vi "get_image_path.vi"(11 "Image directory/path":path) -> (2 "Init image index":u32, 3 "Image path array":path[](array[path]))   [LabVIEW 2024]
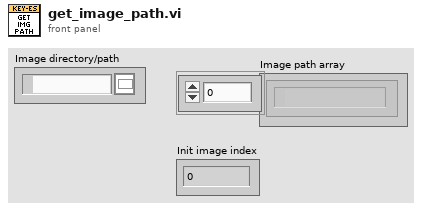
[diagram p1: front panel]
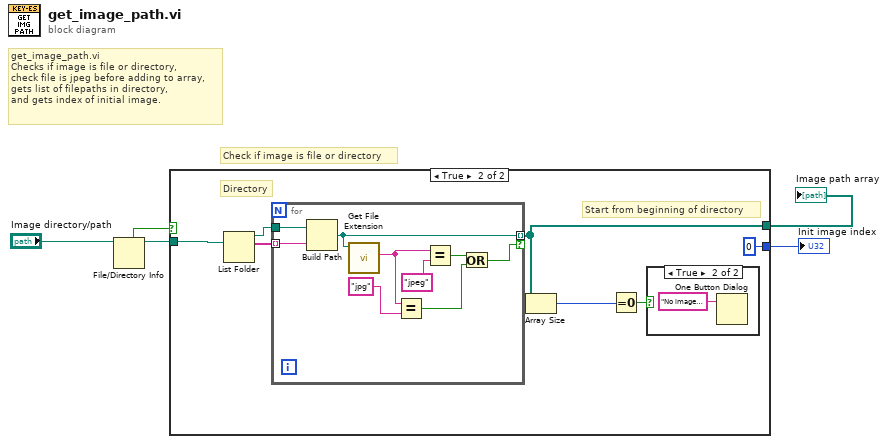
[diagram p0: block diagram]
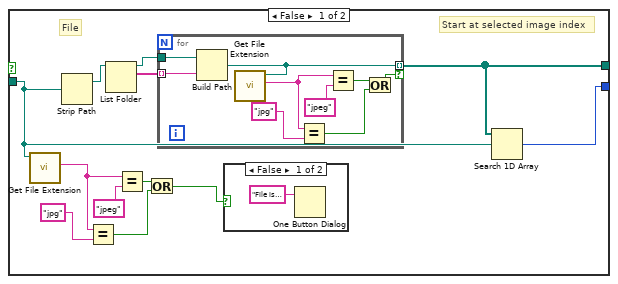
[diagram p2: hidden frame]
diagram:
  # "get_image_path.vi\nChecks if image is file or directory,\ncheck file is jpeg before adding to array,\ngets list of filepaths in directory,\nand gets index of initial image."
  # "Check if image is file or directory"
  n1 = File/Directory Info(path="Image directory/path") -> (path out=w4:path, directory=w5:bool)  [unwired: 1 in, 5 out]
  n2 = case shown="True" w5 {
    tunnel: w4 -> [w14 w34]
    tunnel: [w13 w30] -> w2
    tunnel: [w12 u32 0 ("millisecond multiple")] -> w1
    frame False {
      # "File"
      # "Start at selected image index"
      n3 = call <vilib>:"Get File Extension.vi"("file"=w14) -> ("lowercase file extension"=w7:string)  [unwired: 6 in, 4 out]
      n4 = Strip Path(path=w14) -> (stripped path=w15:path)  [unwired: 1 out]
      n5 = Equal?(x=w7, y="jpg") -> (x = y?=w9:bool)
      n6 = List Folder(path=w15) -> (path out=w16:path, filenames=w17:string[])  [unwired: 3 in, 2 out]
      n7 = Equal?(x=w7, y="jpeg") -> (x = y?=w10:bool)
      n8 = Or(x=w10, y=w9) -> (x .or. y?=w6:bool)
      n9 = for {
        tunnel: w17 -> [w25] mode=indexing
        tunnel: w16 -> [w26]
        tunnel: [w24] -> w13 mode=indexing if=w18
        n10 = Build Path(base path=w26, name or relative path=w25) -> (appended path=w24:path)
        n11 = call <vilib>:"Get File Extension.vi"("file"=w24) -> ("lowercase file extension"=w19:string)  [unwired: 6 in, 4 out]
        n12 = Equal?(x=w19, y="jpg") -> (x = y?=w21:bool)
        n13 = Equal?(x=w19, y="jpeg") -> (x = y?=w22:bool)
        n14 = Or(x=w22, y=w21) -> (x .or. y?=w18:bool)
      }
      n15 = case shown="False" w6 {
        frame False {
          n16 = One Button Dialog(message="File is not an image.") -> ()  [unwired: 1 in, 1 out]
        }
        frame True {
        }
      }
      n17 = Search 1D Array(1D array=w13, element=w14) -> (index of element=w12:i32)  [unwired: 1 in]
    }
    frame True {
      # "Directory"
      # "Start from beginning of directory"
      n18 = List Folder(path=w34) -> (path out=w32:path, filenames=w33:string[])  [unwired: 3 in, 2 out]
      n19 = for {
        tunnel: w33 -> [w44] mode=indexing
        tunnel: w32 -> [w43]
        tunnel: [w42] -> w30 mode=indexing if=w36
        n20 = Build Path(base path=w43, name or relative path=w44) -> (appended path=w42:path)
        n21 = call <vilib>:"Get File Extension.vi"("file"=w42) -> ("lowercase file extension"=w37:string)  [unwired: 6 in, 4 out]
        n22 = Equal?(x=w37, y="jpg") -> (x = y?=w39:bool)
        n23 = Equal?(x=w37, y="jpeg") -> (x = y?=w40:bool)
        n24 = Or(x=w40, y=w39) -> (x .or. y?=w36:bool)
      }
      n25 = Array Size(array=w30) -> (size(s)=w29:i32)
      n26 = Equal To 0?(x=w29) -> (x = 0?=w28:bool)
      n27 = case shown="True" w28 {
        frame False {
        }
        frame True {
          n28 = One Button Dialog(message="No images found in directory.") -> ()  [unwired: 1 in, 1 out]
        }
      }
    }
  }
  "Init image index" <- w1
  "Image path array" <- w2
